vi "핑어연동시험.vi"() -> (0 "불리언 2":bool)   [LabVIEW 2017]
uses:
  <vilib>/Instr/_visa.llb/VISA Configure Serial Port (Instr).vi
panel:
  in  "pwm 주파수":bool
  in  "PWM  주파수":dbl
  in  "COM포트":refnum<visa-resource-name>
  out "Rx":string
  out "Tx":string
  out "PLC REQ":bool
  in  "PNG OFF":bool
  out "종료":bool
  out "PNG OFF":bool
  in  "종료":bool
  out "PNG ON":bool
  in  "PNG ON":bool
  in  "PLC 요청":bool
  # "AUV Pinger TEST"
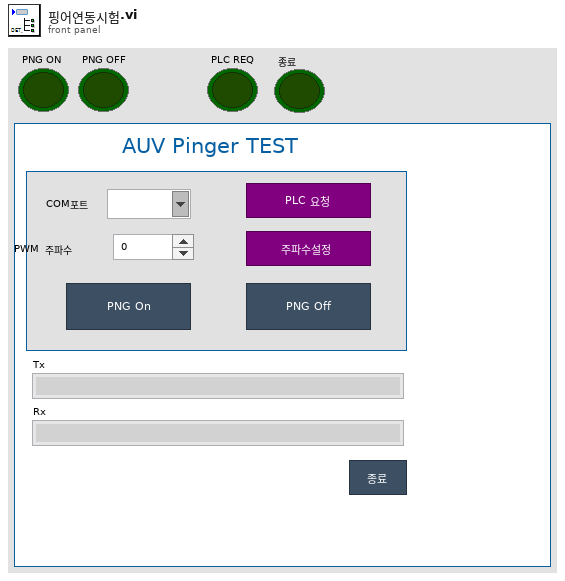
[diagram p1: front panel]
types:
  T1 = enum16{"Init", "Wait", "PLC요청", "PNG ON", "PNG OFF", "PWM Freq", "Stop"}
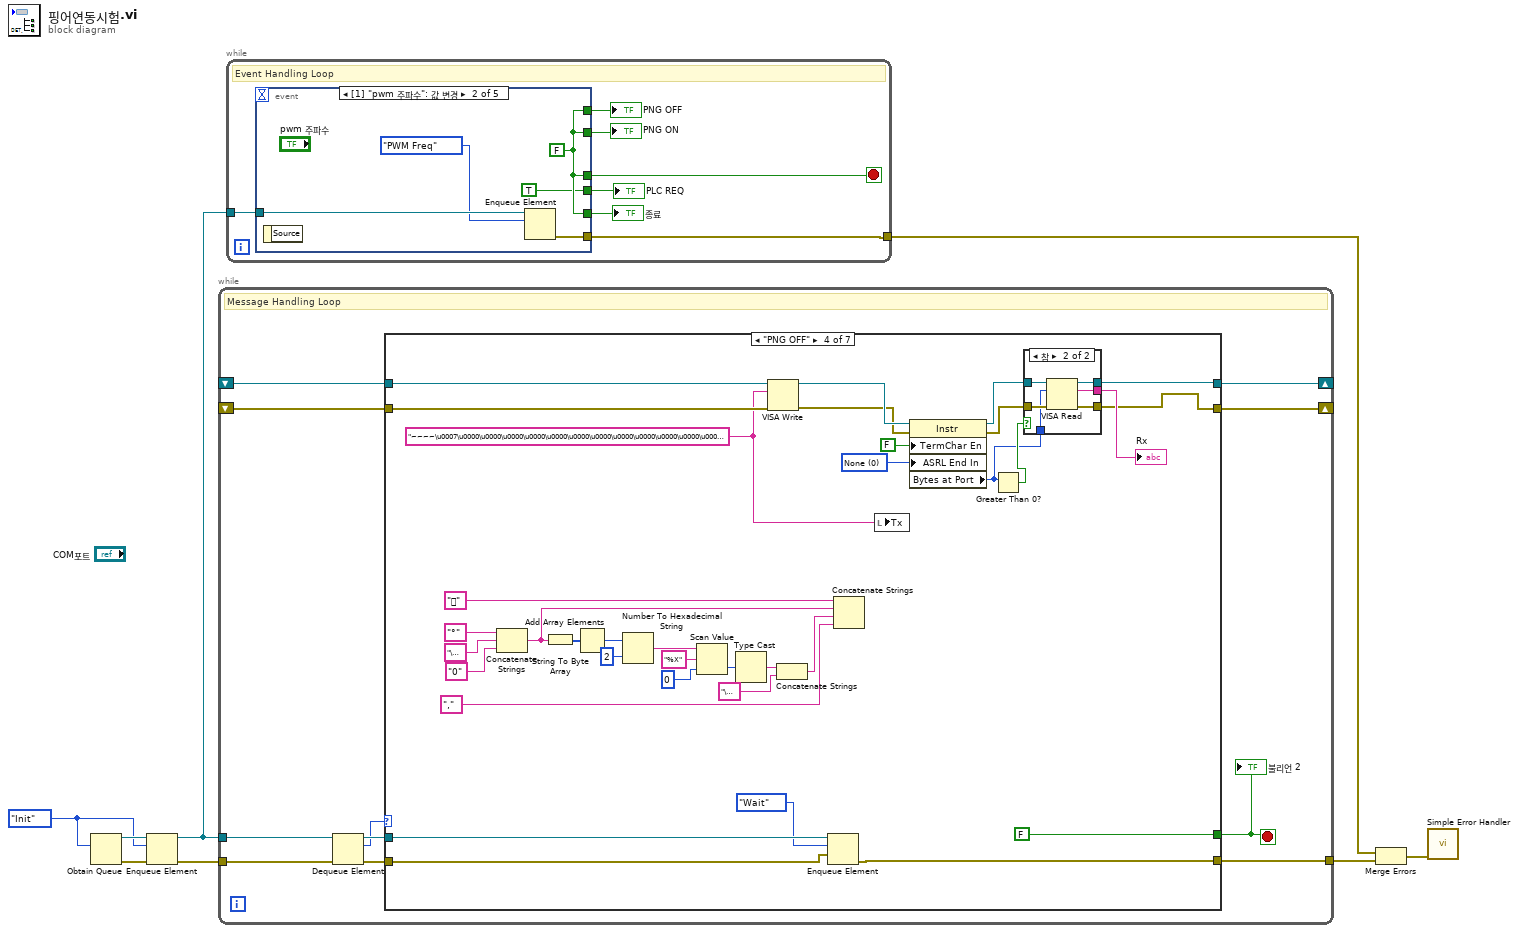
[diagram p0: block diagram]
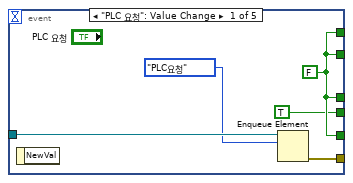
[diagram p2: hidden frame]
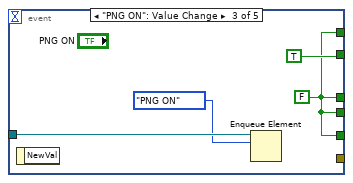
[diagram p3: hidden frame]
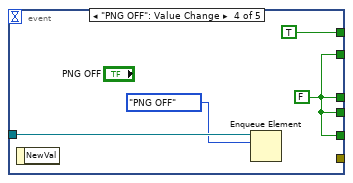
[diagram p4: hidden frame]
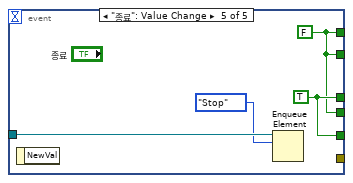
[diagram p5: hidden frame]
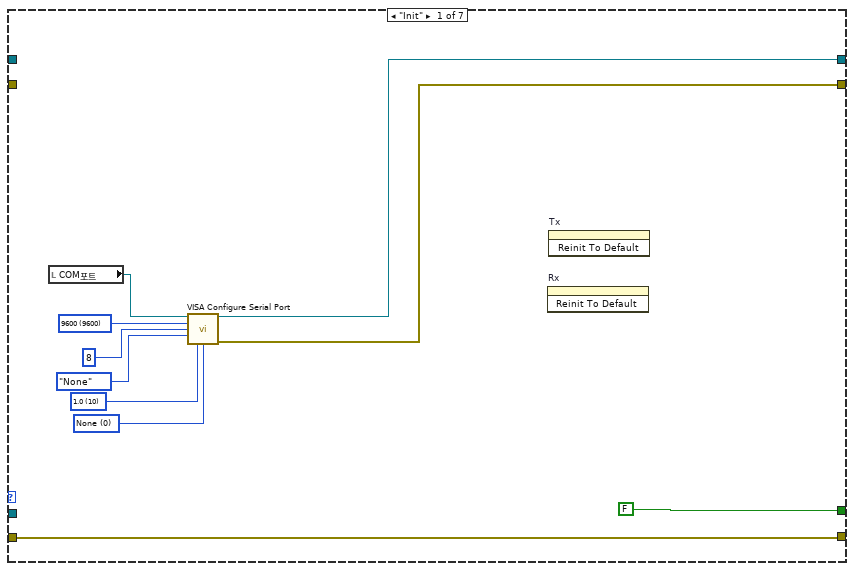
[diagram p6: hidden frame]
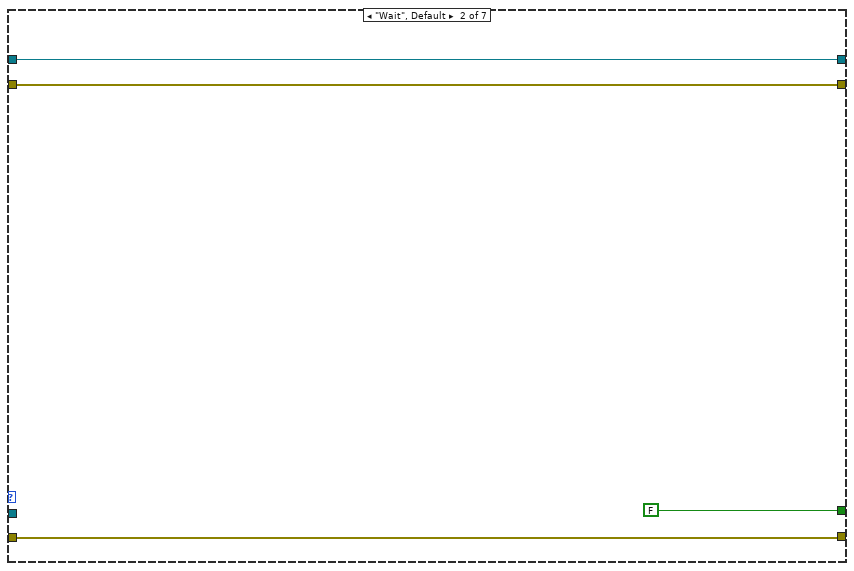
[diagram p7: hidden frame]
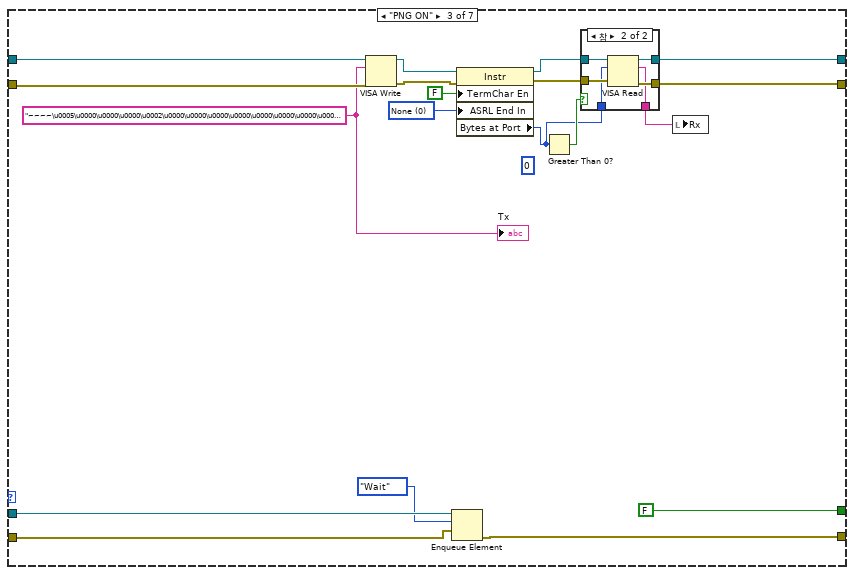
[diagram p8: hidden frame]
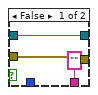
[diagram p9: hidden frame]
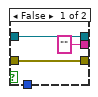
[diagram p10: hidden frame]
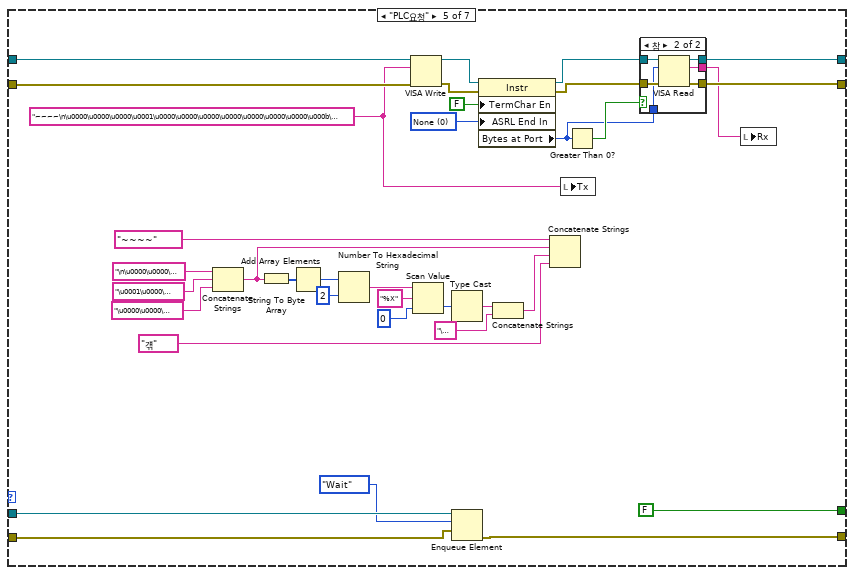
[diagram p11: hidden frame]
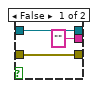
[diagram p12: hidden frame]
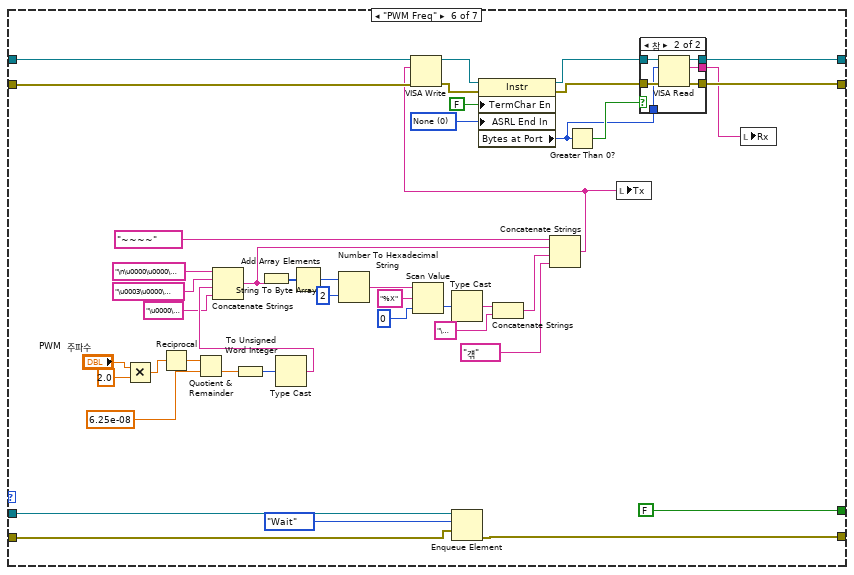
[diagram p13: hidden frame]
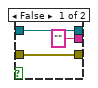
[diagram p14: hidden frame]
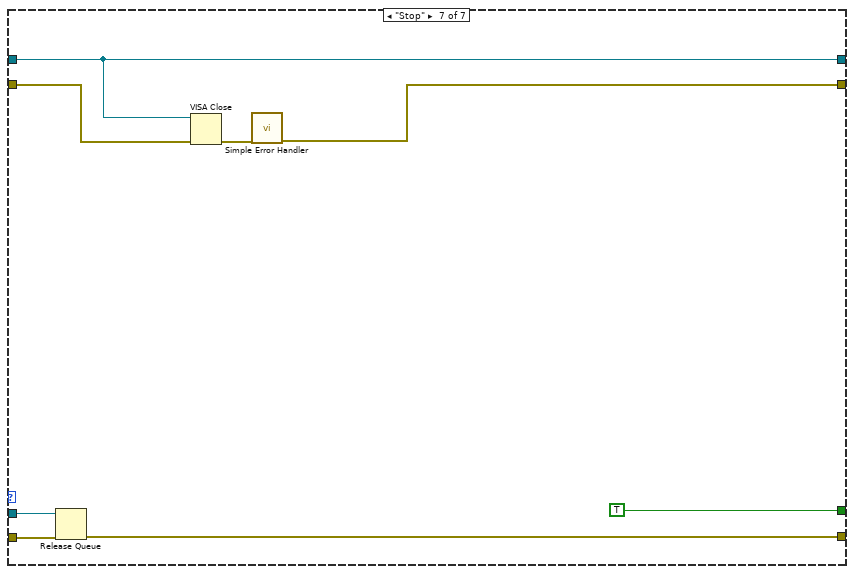
[diagram p15: hidden frame]
diagram:
  w4 = T1."Init" ("열거형")
  n1 = Obtain Queue(element data type=w4) -> (queue out=w7:refnum<queue>, error out=w8:errorcluster)  [unwired: 4 in, 1 out]
  n2 = Enqueue Element(queue=w7, element=w4, error in (no error)=w8) -> (queue out=w5:refnum<queue>, error out=w6:errorcluster)  [unwired: 1 in, 1 out]
  n3 = while {
    tunnel: w5 -> [w18]
    tunnel: w6 -> [w19]
    tunnel: [w14] -> w3
    shift-right: [w12] -> _
    shift-left: _ -> [w11]
    shift-right: [w10] -> _
    shift-left: _ -> [w9]
    stop <- w13 stop-if-true
    # "Message Handling Loop"
    n4 = Dequeue Element(queue=w18, error in (no error)=w19) -> (queue out=w17:refnum<queue>, element=w15:T1, error out=w16:errorcluster)  [unwired: 1 in, 1 out]
    n5 = case "Message Cases" shown="\"PNG OFF\"" w15 {
      tunnel: w17 -> [_ _ w52 w96 w140 w192 w208]
      tunnel: w16 -> [w29 w33 w51 w95 w139 w191 w207]
      tunnel: [w29 w33 w50 w94 w138 w190 w206] -> w14
      tunnel: [FALSE FALSE FALSE FALSE FALSE FALSE TRUE] -> w13
      tunnel: [w27 w31 w46 w67 w118 w171 w205] -> w12
      tunnel: w11 -> [_ w31 w48 w92 w136 w188 w205]
      tunnel: [w21 w30 w45 w66 w117 w170 w202] -> w10
      tunnel: w9 -> [_ w30 w47 w91 w135 w187 w204]
      frame "Init" {
        w22 = u16 0 items=["None"=0, "XON/XOFF"=1, "RTS/CTS"=2, "DTR/DSR"=4] ("flow control")
        w23 = u16 10 items=["1.0"=10, "1.5"=15, "2.0"=20] ("stop bits")
        w26 = u32 9600 items=["75"=75, "110"=110, "134"=134, "150"=150, "300"=300, "600"=600, "1200"=1200, "1800"=1800, "2400"=2400, "4800"=4800, "7200"=7200, "9600"=9600, "14400"=14400, "19200"=19200, "28800"=28800, "38400"=38400, "56000"=56000, "57600"=57600, "115200"=115200, "128000"=128000, "230400"=230400] ("baud rate")
        (unwired) "Init"
        (unwired) FALSE
        (unwired) "Init"
        # "Initialize - Perform any initialization code for your application here. In this example, the only initialization required is setting the Display Message indicator value to an empty string."
        n6 = local read "COM포트"() -> (w20:refnum<visa-resource-name>)
        n7 = call-poly "VISA Configure Serial Port"("VISA resource name"=w20, "baud rate (9600)"=w26, "data bits (8)"=u16 8 ("data bits"), "parity (0:none)"=enum16{"None", "Odd", "Even", "Mark", "Space"}."None" ("parity"), "stop bits (10: 1 bit)"=w23, "flow control (0:none)"=w22) -> ("VISA resource name out"=w27:refnum<visa-resource-name>, "error out"=w21:errorcluster)  [unwired: 3 in, 5 out]
        n8 = invoke on="Rx" class="Str" method="Reinit To Default"() -> ()  [unwired: 3 in, 3 out]
        n9 = invoke on="Tx" class="Str" method="Reinit To Default"() -> ()  [unwired: 3 in, 3 out]
      }
      frame "Wait", Default {
      }
      frame "PNG ON" {
        (unwired) u32 0 ("바이트 카운트")
        w42 = u16 0 items=["None", "Last Bit", "TermChar"] ("Serial Settings:End Mode for Reads")
        w37 = "~~~~\u0005\u0000\u0000\u0000\u0002\u0000\u0000\u0000\u0000\u0000\u0000\u0000\u0007\u0000" ("Tx")
        (unwired) "역방향"
        # "Action 2 - Send an \"Update Display\" message indicating which button was pressed. Note that a string is sent as the Message Data along with the \"Update Display\" message."
        n10 = VISA Write(VISA resource name=w48, write buffer=w37, error in (no error)=w47) -> (VISA resource name out=w41:refnum<visa-resource-name>, error out=w40:errorcluster)  [unwired: 1 out]
        n11 = Enqueue Element(queue=w52, element=T1."Wait" ("열거형"), error in (no error)=w51) -> (error out=w50:errorcluster)  [unwired: 1 in, 2 out]
        n12 = property class="Instr"(reference=w41, error in=w40, "TermChar En"=FALSE ("Message Based Settings:Termination Character Enable"), "ASRL End In"=w42) -> (reference out=w39:refnum<visa-resource-name>, error out=w38:errorcluster, "Bytes at Port"=w35:u32)
        n13 = Greater Than 0?(x=w35) -> (x > 0?=w36:bool)
        n14 = case shown="참" w36 {
          tunnel: [w55 w61] -> w46
          tunnel: [w54 w60] -> w45
          tunnel: ["" ("read buffer") w59] -> w44
          tunnel: w39 -> [w55 w58]
          tunnel: w38 -> [w54 w57]
          tunnel: w35 -> [_ w56]
          frame False {
          }
          frame True {
            n15 = VISA Read(VISA resource name=w58, byte count=w56, error in (no error)=w57) -> (VISA resource name out=w61:refnum<visa-resource-name>, read buffer=w59:string, error out=w60:errorcluster)  [unwired: 1 out]
          }
        }
        n16 = local write "Rx"(w44) -> ()
        "Tx" <- w37
      }
      frame "PNG OFF" {
        w68 = u16 0 items=["None", "Last Bit", "TermChar"] ("Serial Settings:End Mode for Reads")
        w65 = "~~~~\u0007\u0000\u0000\u0000\u0000\u0000\u0000\u0000\u0000\u0000\u0000\u0000\u0007\u0000" ("Tx")
        (unwired) "역방향"
        # "Action 2 - Send an \"Update Display\" message indicating which button was pressed. Note that a string is sent as the Message Data along with the \"Update Display\" message."
        n17 = Concatenate Strings("°" ("문자열"), "\u0001" ("문자열"), "0" ("버퍼 쓰기")) -> (w80:string)
        n18 = String To Byte Array(string=w80) -> (unsigned byte array=w87:u8[])
        n19 = Add Array Elements(numeric array=w87) -> (sum=w85:u8)
        n20 = Number To Hexadecimal String(1:i16 2 ("폭(-)"), 2:w85) -> (0:w83:string)
        n21 = Scan Value(string=w83, format string="%X" ("포맷 문자열"), default (0 dbl)=u8 0 ("기본(0 dbl)")) -> (value=w82:u8)  [unwired: 1 out]
        n22 = Type Cast(x=w82) -> (*(type *) &x=w77:string)  [unwired: 1 in]
        n23 = VISA Write(VISA resource name=w92, write buffer=w65, error in (no error)=w91) -> (VISA resource name out=w73:refnum<visa-resource-name>, error out=w72:errorcluster)  [unwired: 1 out]
        n24 = Concatenate Strings(w77, "\u0000" ("버퍼 쓰기")) -> (w75:string)
        n25 = Enqueue Element(queue=w96, element=T1."Wait" ("열거형"), error in (no error)=w95) -> (error out=w94:errorcluster)  [unwired: 1 in, 2 out]
        n26 = Concatenate Strings("" ("버퍼 쓰기"), w80, w75, "‚" ("버퍼 쓰기")) -> ()  [unwired: 1 out]
        n27 = local write "Tx"(w65) -> ()
        n28 = property class="Instr"(reference=w73, error in=w72, "TermChar En"=FALSE ("Message Based Settings:Termination Character Enable"), "ASRL End In"=w68) -> (reference out=w71:refnum<visa-resource-name>, error out=w70:errorcluster, "Bytes at Port"=w63:u32)
        n29 = Greater Than 0?(x=w63) -> (x > 0?=w64:bool)
        n30 = case shown="참" w64 {
          tunnel: ["" ("read buffer") w105] -> w74
          tunnel: w71 -> [w99 w104]
          tunnel: w70 -> [w98 w103]
          tunnel: [w99 w102] -> w67
          tunnel: [w98 w101] -> w66
          tunnel: w63 -> [_ w100]
          frame False {
          }
          frame True {
            n31 = VISA Read(VISA resource name=w104, byte count=w100, error in (no error)=w103) -> (VISA resource name out=w102:refnum<visa-resource-name>, read buffer=w105:string, error out=w101:errorcluster)  [unwired: 1 out]
          }
        }
        "Rx" <- w74
      }
      frame "PLC요청" {
        w114 = u16 0 items=["None", "Last Bit", "TermChar"] ("Serial Settings:End Mode for Reads")
        w109 = "~~~~\n\u0000\u0000\u0000\u0001\u0000\u0000\u0000\u0000\u0000\u0000\u0000\u000b\u0000" ("Tx")
        (unwired) "역방향"
        # "Action 2 - Send an \"Update Display\" message indicating which button was pressed. Note that a string is sent as the Message Data along with the \"Update Display\" message."
        n32 = Concatenate Strings("\n\u0000\u0000\u0000" ("문자열"), "\u0001\u0000\u0000\u0000" ("문자열"), "\u0000\u0000\u0000\u0000" ("버퍼 쓰기")) -> (w124:string)
        n33 = String To Byte Array(string=w124) -> (unsigned byte array=w131:u8[])
        n34 = Add Array Elements(numeric array=w131) -> (sum=w129:u8)
        n35 = Number To Hexadecimal String(1:i16 2 ("폭(-)"), 2:w129) -> (0:w127:string)
        n36 = VISA Write(VISA resource name=w136, write buffer=w109, error in (no error)=w135) -> (VISA resource name out=w113:refnum<visa-resource-name>, error out=w112:errorcluster)  [unwired: 1 out]
        n37 = Scan Value(string=w127, format string="%X" ("포맷 문자열"), default (0 dbl)=u8 0 ("기본(0 dbl)")) -> (value=w126:u8)  [unwired: 1 out]
        n38 = Type Cast(x=w126) -> (*(type *) &x=w121:string)  [unwired: 1 in]
        n39 = Enqueue Element(queue=w140, element=T1."Wait" ("열거형"), error in (no error)=w139) -> (error out=w138:errorcluster)  [unwired: 1 in, 2 out]
        n40 = property class="Instr"(reference=w113, error in=w112, "TermChar En"=FALSE ("Message Based Settings:Termination Character Enable"), "ASRL End In"=w114) -> (reference out=w111:refnum<visa-resource-name>, error out=w110:errorcluster, "Bytes at Port"=w107:u32)
        n41 = Concatenate Strings(w121, "\u0000" ("버퍼 쓰기")) -> (w119:string)
        n42 = Concatenate Strings("~~~~" ("버퍼 쓰기"), w124, w119, "걖" ("버퍼 쓰기")) -> ()  [unwired: 1 out]
        n43 = local write "Tx"(w109) -> ()
        n44 = Greater Than 0?(x=w107) -> (x > 0?=w108:bool)
        n45 = case shown="참" w108 {
          tunnel: [w143 w149] -> w118
          tunnel: [w142 w148] -> w117
          tunnel: ["" ("read buffer") w147] -> w116
          tunnel: w111 -> [w143 w146]
          tunnel: w110 -> [w142 w145]
          tunnel: w107 -> [_ w144]
          frame False {
          }
          frame True {
            n46 = VISA Read(VISA resource name=w146, byte count=w144, error in (no error)=w145) -> (VISA resource name out=w149:refnum<visa-resource-name>, read buffer=w147:string, error out=w148:errorcluster)  [unwired: 1 out]
          }
        }
        n47 = local write "Rx"(w116) -> ()
      }
      frame "PWM Freq" {
        w167 = u16 0 items=["None", "Last Bit", "TermChar"] ("Serial Settings:End Mode for Reads")
        (unwired) "역방향"
        # "Action 2 - Send an \"Update Display\" message indicating which button was pressed. Note that a string is sent as the Message Data along with the \"Update Display\" message."
        n48 = Multiply(x="PWM  주파수", y=2.0) -> (x*y=w156:dbl)
        n49 = Reciprocal(x=w156) -> (1/x=w160:dbl)
        n50 = Quotient & Remainder(x=w160, y=6.25e-08) -> (floor(x/y)=w153:dbl)  [unwired: 1 out]
        n51 = To Unsigned Word Integer(number=w153) -> (unsigned 16bit integer=w152:u16)
        n52 = Type Cast(x=w152) -> (*(type *) &x=w151:string)  [unwired: 1 in]
        n53 = Concatenate Strings("\n\u0000\u0000\u0000" ("문자열"), "\u0003\u0000\u0000\u0000" ("문자열"), w151, "\u0000\u0000" ("버퍼 쓰기")) -> (w177:string)
        n54 = String To Byte Array(string=w177) -> (unsigned byte array=w184:u8[])
        n55 = Add Array Elements(numeric array=w184) -> (sum=w182:u8)
        n56 = Number To Hexadecimal String(1:i16 2 ("폭(-)"), 2:w182) -> (0:w180:string)
        n57 = Scan Value(string=w180, format string="%X" ("포맷 문자열"), default (0 dbl)=u8 0 ("기본(0 dbl)")) -> (value=w179:u8)  [unwired: 1 out]
        n58 = Type Cast(x=w179) -> (*(type *) &x=w174:string)  [unwired: 1 in]
        n59 = Enqueue Element(queue=w192, element=T1."Wait" ("열거형"), error in (no error)=w191) -> (error out=w190:errorcluster)  [unwired: 1 in, 2 out]
        n60 = Concatenate Strings(w174, "\u0000" ("버퍼 쓰기")) -> (w172:string)
        n61 = Concatenate Strings("~~~~" ("버퍼 쓰기"), w177, w172, "걖" ("버퍼 쓰기")) -> (w155:string)
        n62 = VISA Write(VISA resource name=w188, write buffer=w155, error in (no error)=w187) -> (VISA resource name out=w166:refnum<visa-resource-name>, error out=w165:errorcluster)  [unwired: 1 out]
        n63 = property class="Instr"(reference=w166, error in=w165, "TermChar En"=FALSE ("Message Based Settings:Termination Character Enable"), "ASRL End In"=w167) -> (reference out=w164:refnum<visa-resource-name>, error out=w163:errorcluster, "Bytes at Port"=w161:u32)
        n64 = Greater Than 0?(x=w161) -> (x > 0?=w162:bool)
        n65 = local write "Tx"(w155) -> ()
        n66 = case shown="참" w162 {
          tunnel: [w195 w201] -> w171
          tunnel: [w194 w200] -> w170
          tunnel: ["" ("read buffer") w199] -> w169
          tunnel: w164 -> [w195 w198]
          tunnel: w163 -> [w194 w197]
          tunnel: w161 -> [_ w196]
          frame False {
          }
          frame True {
            n67 = VISA Read(VISA resource name=w198, byte count=w196, error in (no error)=w197) -> (VISA resource name out=w201:refnum<visa-resource-name>, read buffer=w199:string, error out=w200:errorcluster)  [unwired: 1 out]
          }
        }
        n68 = local write "Rx"(w169) -> ()
      }
      frame "Stop" {
        n69 = Release Queue(queue=w208, error in (no error)=w207) -> (error out=w206:errorcluster)  [unwired: 1 in, 2 out]
        n70 = VISA Close(VISA resource name=w205, error in (no error)=w204) -> (error out=w203:errorcluster)
        n71 = call <vilib>:"Simple Error Handler.vi"("error in (no error)"=w203) -> ("error out"=w202:errorcluster)  [unwired: 1 in, 7 out]
      }
    }
    "불리언 2" <- w13
  }
  n72 = while {
    tunnel: w5 -> [w216]
    tunnel: [w215] -> w2
    stop <- w214 stop-if-true
    # "Event Handling Loop"
    n73 = event shown="[1] \"pwm 주파수\": 값 변경" {
      selector: _ -> [_ _ _ _ _]
      dyn-events: _ -> [_ _ _ _ _]
      timeout: _ -> [_ _ _ _ _]
      tunnel: w216 -> [w221 w226 w230 w234 w238]
      tunnel: [w220 w225 _ _ _] -> w215
      tunnel: [w219 w224 w228 w232 w237] -> w214
      tunnel: [w219 w224 TRUE w232 w236] -> w212
      tunnel: [w219 w224 w228 TRUE w236] -> w213
      tunnel: [w219 w224 w228 w232 w237] -> w211
      tunnel: [TRUE TRUE w228 w232 w236] -> w210
      event "PLC 요청": Value Change {
        w219 = FALSE
        # "Enqueue an \"Action 2\" message."
        n74 = event-data() -> ()  [unwired: 1 in, 1 out]
        n75 = Enqueue Element(queue=w221, element=T1."PLC요청" ("열거형")) -> (error out=w220:errorcluster)  [unwired: 2 in, 2 out]
      }
      event "pwm 주파수": Value Change {
        w224 = FALSE
        # "Enqueue an \"Action 2\" message."
        n76 = event-data() -> ()  [unwired: 1 in, 1 out]
        n77 = Enqueue Element(queue=w226, element=T1."PWM Freq" ("열거형")) -> (error out=w225:errorcluster)  [unwired: 2 in, 2 out]
      }
      event "PNG ON": Value Change {
        w228 = FALSE
        n78 = event-data() -> ()  [unwired: 1 in, 1 out]
        n79 = Enqueue Element(queue=w230, element=T1."PNG ON" ("열거형")) -> ()  [unwired: 2 in, 3 out]
      }
      event "PNG OFF": Value Change {
        w232 = FALSE
        n80 = event-data() -> ()  [unwired: 1 in, 1 out]
        n81 = Enqueue Element(queue=w234, element=T1."PNG OFF" ("열거형")) -> ()  [unwired: 2 in, 3 out]
      }
      event "종료": Value Change {
        w236 = FALSE
        w237 = TRUE
        n82 = event-data() -> ()  [unwired: 1 in, 1 out]
        n83 = Enqueue Element(queue=w238, element=T1."Stop" ("열거형")) -> ()  [unwired: 2 in, 3 out]
      }
    }
    "PNG ON" <- w212
    "PNG OFF" <- w213
    "종료" <- w211
    "PLC REQ" <- w210
  }
  n84 = Merge Errors(w2, w3) -> (w1:errorcluster)
  n85 = call <vilib>:"Simple Error Handler.vi"("error in (no error)"=w1) -> ()  [unwired: 4 in, 5 out]
